vi "ROS_Master_GetPubSubUnsubscribe.vi"(2 "Value":string, 3 "String w/o Tag":string) -> (0 "Direction":enum16{"Publisher", "Subscriber"}(ring)=enum."Subscriber", 1 "PubSub":T1)   [LabVIEW 2016]
doc: "Takes an XML string for unregistering a publisher and subscriber and returns a cluster of\n-Topic\n-IP\n-Caller ID"
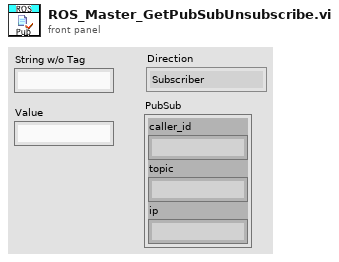
[diagram p1: front panel]
types:
  T1 = cluster{"caller_id":string, "topic":string, "ip":string}
  T2 = cluster{"value":string, "value":string, "value":string}
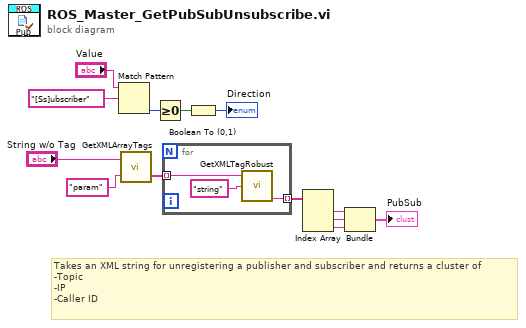
[diagram p0: block diagram]
diagram:
  # "Takes an XML string for unregistering a publisher and subscriber and returns a cluster of\n-Topic\n-IP\n-Caller ID"
  n1 = Match Pattern(string="Value", regular expression="[Ss]ubscriber") -> (offset past match=w10:i32)  [unwired: 1 in, 3 out]
  n2 = call "GetXMLArrayTags.vi"("ArrayTag"="param", "String"="String w/o Tag") -> ("Array"=w3:string[])  [unwired: 1 out]
  n3 = Greater Or Equal To 0?(x=w10) -> (x >= 0?=w11:bool)
  n4 = for {
    tunnel: w3 -> [w16] mode=indexing
    tunnel: [w14] -> w4 mode=indexing
    n5 = call "GetXMLTagRobust.vi"("Tag"="string", "String"=w16) -> ("value"=w14:string)  [unwired: 1 in, 3 out]
  }
  n6 = Boolean To (0,1)(Boolean=w11) -> (0, 1=→"Direction":i16)
  n7 = Index Array(array=w4) -> (element #1=w5:string, element #2=w6:string, element #3=w7:string)  [unwired: 3 in]
  n8 = Bundle("value"=w5, "value"=w6, "value"=w7) -> (→"PubSub":T2)  [unwired: 1 in]
